vi "Test_WriteValue_CheckCaption_CaptionUpdated.vi"(8 "error in (no error)":errorcluster, 11 "TestCase in":refnum<class "TestTerminalCaptionBinding.lvclass">) -> (0 "error out":errorcluster, 3 "TestCase out":refnum<class "TestTerminalCaptionBinding.lvclass">)   [LabVIEW 2017, in "TestTerminalCaptionBinding.lvclass"]
uses:
  TestTerminalCaptionBinding.lvclass
  Source/Concrete/TerminalCaptionBinding/TerminalCaptionBinding.lvclass
  C:/Git/composed-transport/Source/ITransport/ITransport.lvclass
  Source/ITransport/ITransport.lvclass
panel:
  in  "Numeric":i32 caption="A"
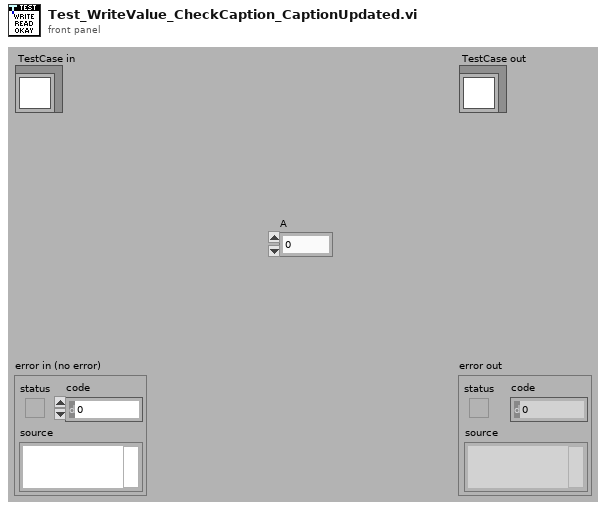
[diagram p1: front panel]
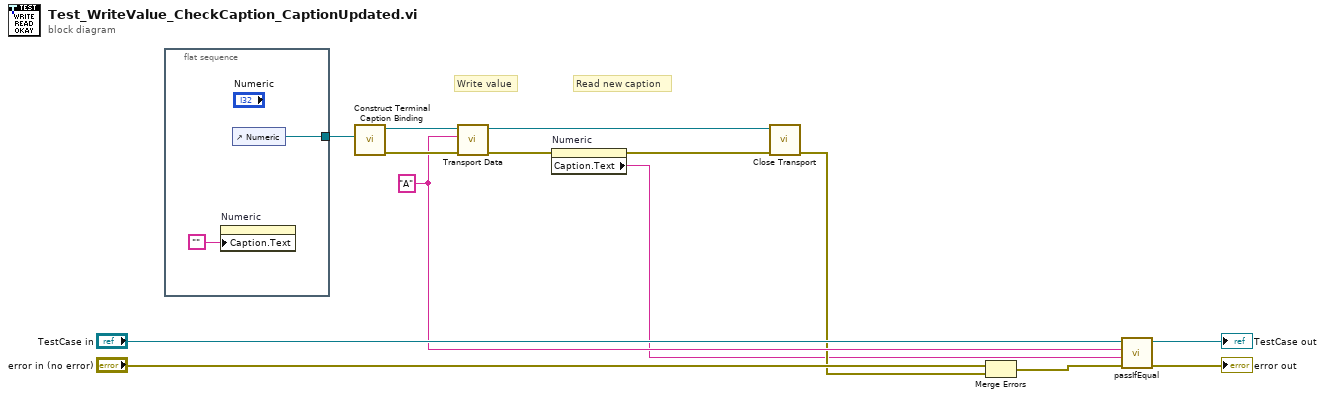
[diagram p0: block diagram]
diagram:
  w4 = "A"
  # "Read new caption"
  # "Write value"
  n1 = flat-sequence {
    tunnel: [w16] -> w6
    frame #0 {
      n2 = property on="Numeric" class="DigNum (strict)"("Caption.Text"="") -> ()  [unwired: 2 in, 2 out]
      n3 = control-ref of="Numeric"() -> (w16:refnum<vi>)
    }
  }
  n4 = call "Construct Terminal Caption Binding.vi"("Ctl Refnum"=w6) -> ("error out"=w14:errorcluster, "TerminalCaptionBinding"=w9:refnum<class "TerminalCaptionBinding.lvclass">)  [unwired: 9 in]
  n5 = call "Transport Data.vi"("error in (no error)"=w14, "Value"=w4, "ITransport in"=w9) -> ("error out"=w5:errorcluster, "ITransport out"=w7:refnum<class "TerminalCaptionBinding.lvclass">)  [unwired: 7 in]
  n6 = property on="Numeric" class="DigNum (strict)"(error in=w5) -> (error out=w2:errorcluster, "Caption.Text"=w1:string)  [unwired: 1 in, 1 out]
  n7 = call-dynamic "Close Transport.vi"("error in (no error)"=w2, "ITransport in"=w7) -> ("error out"=w3:errorcluster)  [unwired: 9 in]
  n8 = Merge Errors("error in (no error)", w3) -> (w8:errorcluster)
  n9 = call-dynamic "passIfEqual.vi"("error in (no error)"=w8, "y"=w1, "x"=w4, "TestCase in"="TestCase in") -> ("error out"=→"error out":errorcluster, "TestCase out"=→"TestCase out":refnum<class "TestTerminalCaptionBinding.lvclass">)  [unwired: 6 in]
